vi "Stop Core.vi"(10 "final error code":i32, 11 "ModelCountsObservations In":refnum<class "ModelTimesNObservations.lvclass">) -> (3 "ModelCountsObservations Out":refnum<class "ModelTimesNObservations.lvclass">)   [LabVIEW 2017, in "BenchmarkObservationRate.lvlib" / "ModelTimesNObservations.lvclass"]
doc: "(<B>Filename</B>: Actor Framework.lvlib:Actor.lvclass:Stop Core.vi)\n\nDefines what the actor does before it stops. Use the <B>final error code</B> input to determine whether the actor shut down in response to an error.\n\nBy default, this method does nothing. A descendant class may override it to define behavior, such as shutting down any processes the actor initiated in its override of the Actor Core method."
uses:
  ModelTimesNObservations.lvclass
  ModelTimesNObservations.lvclass/ModelTimesNObservations.ctl
  Source/IModel/IModel/IModel.lvclass
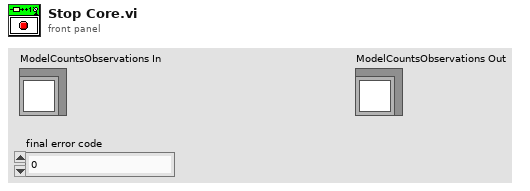
[diagram p1: front panel]
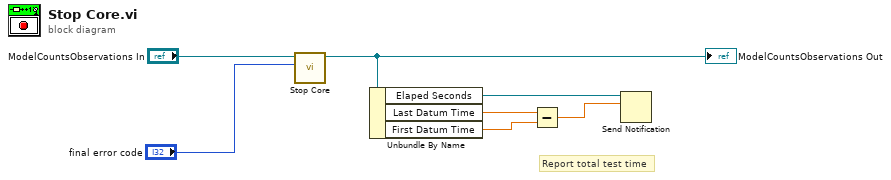
[diagram p0: block diagram]
diagram:
  # "Report total test time"
  n1 = call-parent "Stop Core.vi"("final error code"="final error code", "IObserver in"="ModelCountsObservations In") -> ("IObserver out"=w6:refnum<class "ModelTimesNObservations.lvclass">)  [unwired: 9 in]
  "ModelCountsObservations Out" <- w6
  n2 = Unbundle By Name(w6) -> ("Elaped Seconds"=w5:refnum<notifier>, "Last Datum Time"=w3:dbl, "First Datum Time"=w2:dbl)
  n3 = Subtract(x=w3, y=w2) -> (x-y=w1:dbl)
  n4 = Send Notification(notification=w1, notifier=w5) -> ()  [unwired: 1 in, 2 out]
